vi "find circle corners V3.vi"(7 "method":enum16{"median", "method 2", "histogram"}(ring), 8 "z":cdb[](array[numeric]), 11 "circle corners in":T1={"z (-pi/2)"=-1.0311345636926572+0.5736824521422934i, "z(inf)"=-0.5200164984937075+1.0975277942502903i, "z (pi/2)"=-1.0311345636926572+0.5736824521422934i, "z center"=-0.5136528600391839+0.580046090596817i, "z(0)"=-0.5200164984937075+1.0975277942502903i, "radius"=-1.0311345636926572}) -> (3 "circle corners out":T1={"z (-pi/2)"=-1.0311345636926572+0.5736824521422934i, "z(inf)"=-0.5200164984937075+1.0975277942502903i, "z (pi/2)"=-1.0311345636926572+0.5736824521422934i, "z center"=-0.5136528600391839+0.580046090596817i, "z(0)"=-0.5200164984937075+1.0975277942502903i, "radius"=-1.0311345636926572})   [LabVIEW 2018]
uses:
  circle corners.ctl
  <vilib>/Analysis/baseanly.llb/Mean (DBL).vi
  <vilib>/Analysis/NI_AALBase.lvlib
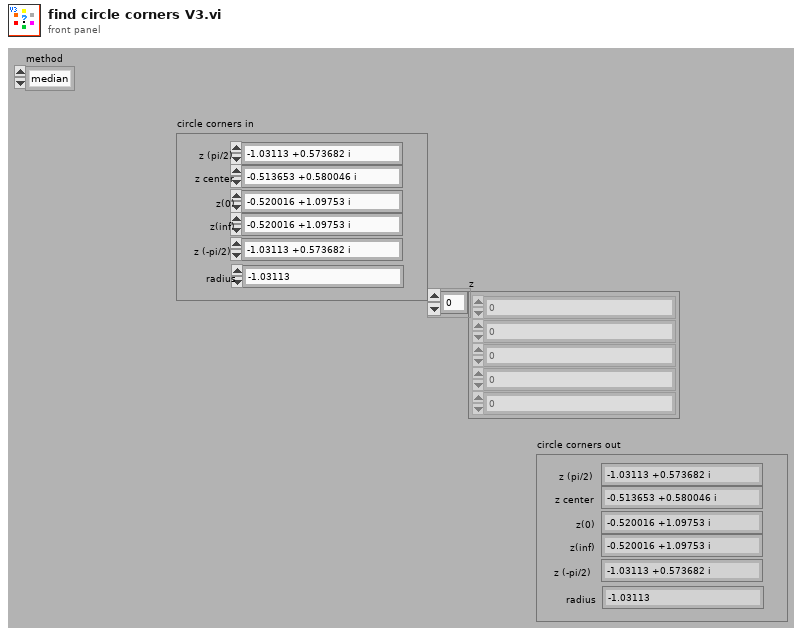
[diagram p1: front panel]
types:
  T1 = typedef "circle corners.ctl" = cluster{"z (-pi/2)":cdb, "z(inf)":cdb, "z (pi/2)":cdb, "z center":cdb, "z(0)":cdb, "radius":dbl}
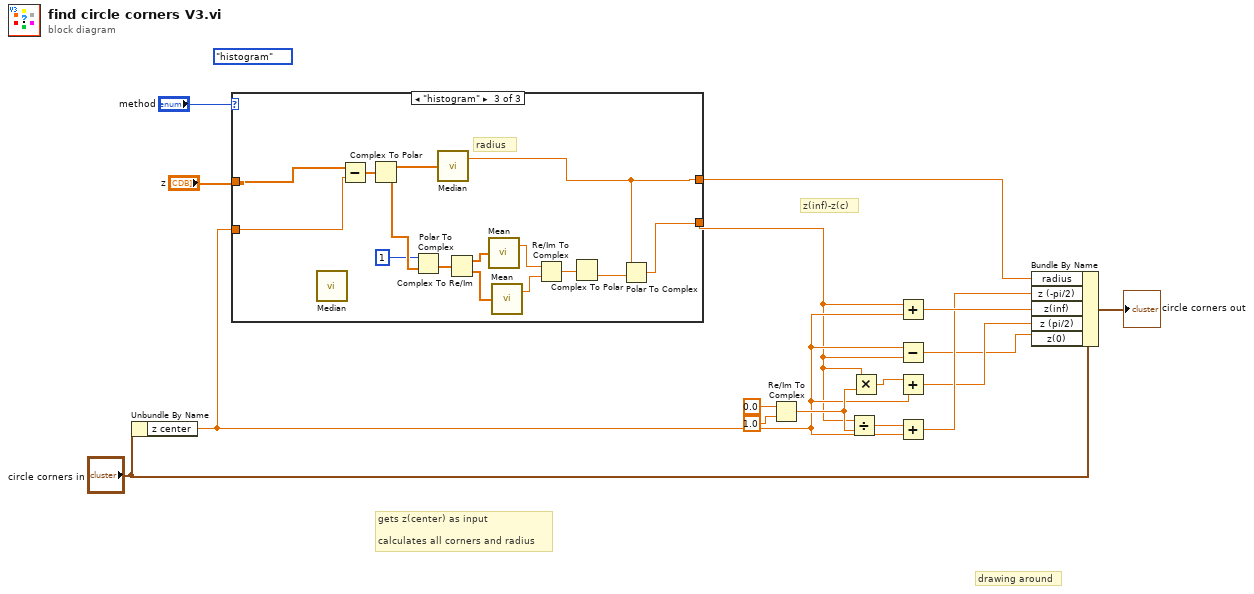
[diagram p0: block diagram]
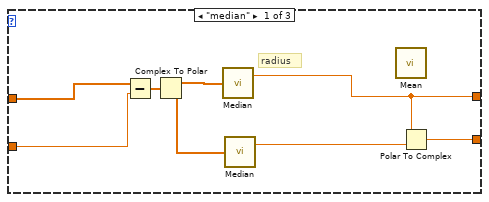
[diagram p2: hidden frame]
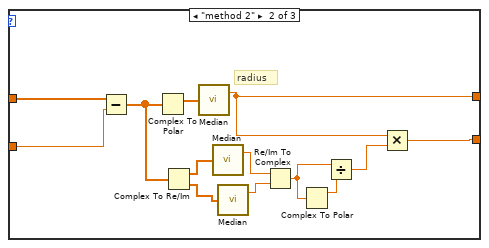
[diagram p3: hidden frame]
diagram:
  (unwired) enum16{"median", "method 2", "histogram"}."histogram"
  # "gets z(center) as input \n\ncalculates all corners and radius"
  # "z(inf)-z(c)"
  # "drawing around"
  n1 = Unbundle By Name("circle corners in") -> ("z center"=w4:cdb)
  n2 = case shown="\"histogram\"" "method" {
    tunnel: "z" -> [w23 w36 w49]
    tunnel: w4 -> [w21 w35 w50]
    tunnel: [w18 w31 w40] -> w5
    tunnel: [w17 w29 w38] -> w2
    frame "median" {
      # "radius"
      n3 = Subtract(x=w23, y=w21) -> (x-y=w24:cdb[])
      n4 = Complex To Polar(r * e^(i*theta)=w24) -> (r=w22:dbl[], theta=w20:dbl[])
      n5 = call <vilib>:"Median.vi"("X"=w22) -> ("median"=w18:dbl)  [unwired: 1 out]
      n6 = call <vilib>:"Median.vi"("X"=w20) -> ("median"=w19:dbl)  [unwired: 1 out]
      n7 = call-poly <vilib>:"Mean.vi"() -> ()  [unwired: 1 in, 2 out]
      n8 = Polar To Complex(1:w19, 2:w18) -> (0:w17:cdb)
    }
    frame "method 2" {
      # "radius"
      n9 = Subtract(x=w36, y=w35) -> (x-y=w34:cdb[])
      n10 = Complex To Polar(r * e^(i*theta)=w34) -> (r=w37:dbl[])  [unwired: 1 out]
      n11 = Complex To Re/Im(x + iy=w34) -> (x=w27:dbl[], y=w28:dbl[])
      n12 = call <vilib>:"Median.vi"("X"=w37) -> ("median"=w31:dbl)  [unwired: 1 out]
      n13 = call <vilib>:"Median.vi"("X"=w27) -> ("median"=w26:dbl)  [unwired: 1 out]
      n14 = call <vilib>:"Median.vi"("X"=w28) -> ("median"=w25:dbl)  [unwired: 1 out]
      n15 = Re/Im To Complex(1:w25, 2:w26) -> (0:w33:cdb)
      n16 = Complex To Polar(r * e^(i*theta)=w33) -> (r=w32:dbl)  [unwired: 1 out]
      n17 = Divide(x=w33, y=w32) -> (x/y=w30:cdb)
      n18 = Multiply(x=w31, y=w30) -> (x*y=w29:cdb)
    }
    frame "histogram" {
      # "radius"
      n19 = call <vilib>:"Median.vi"() -> ()  [unwired: 1 in, 2 out]
      n20 = Subtract(x=w49, y=w50) -> (x-y=w52:cdb[])
      n21 = Complex To Polar(r * e^(i*theta)=w52) -> (r=w51:dbl[], theta=w48:dbl[])
      n22 = Polar To Complex(1:w48, 2:1) -> (0:w46:cdb[])
      n23 = call <vilib>:"Median.vi"("X"=w51) -> ("median"=w40:dbl)  [unwired: 1 out]
      n24 = Complex To Re/Im(x + iy=w46) -> (x=w45:dbl[], y=w44:dbl[])
      n25 = call-poly <vilib>:"Mean.vi"("X"=w45) -> ("mean"=w43:dbl)  [unwired: 1 out]
      n26 = call-poly <vilib>:"Mean.vi"("X"=w44) -> ("mean"=w42:dbl)  [unwired: 1 out]
      n27 = Re/Im To Complex(1:w42, 2:w43) -> (0:w41:cdb)
      n28 = Complex To Polar(r * e^(i*theta)=w41) -> (theta=w39:dbl)  [unwired: 1 out]
      n29 = Polar To Complex(1:w39, 2:w40) -> (0:w38:cdb)
    }
  }
  n30 = Re/Im To Complex(1:1.0 ("y"), 2:0.0 ("x")) -> (0:w12:cdb)
  n31 = Divide(x=w2, y=w12) -> (x/y=w13:cdb)
  n32 = Multiply(x=w2, y=w12) -> (x*y=w14:cdb)
  n33 = Add(x=w2, y=w4) -> (x+y=w11:cdb)
  n34 = Subtract(x=w4, y=w2) -> (x-y=w7:cdb)
  n35 = Add(x=w14, y=w4) -> (x+y=w9:cdb)
  n36 = Add(x=w13, y=w4) -> (x+y=w10:cdb)
  n37 = Bundle By Name(cluster="circle corners in", "radius"=w5, "z (-pi/2)"=w10, "z(inf)"=w11, "z (pi/2)"=w9, "z(0)"=w7) -> (→"circle corners out":T1)
